vi "asap_spectrum.vi"() -> (6 "Raw signal":waveform(dbl)(graph))   [LabVIEW 2013]
uses:
  micron/labview/manipulator/squiggle/Host/i2c_interface.ctl
  micron/labview/manipulator/squiggle/Host/fpga_reference.ctl
  <vilib>/DAQmx/read.llb/DAQmx Read (Analog Wfm 1Chan NSamp).vi
  <vilib>/Analysis/2dsp.llb/Real FFT.vi
  <vilib>/Analysis/2dsp.llb/Inverse Real FFT.vi
  initialization/globals.vi
  <vilib>/DAQmx/miscellaneous.llb/DAQmx Fill In Error Info.vi
  <vilib>/Waveform/WDTOps.llb/WDT Get Waveform Subset DBL.vi
  <vilib>/Analysis/NI_AALPro.lvlib
panel:
  in  "Noise":bool
  out "Residue":waveform(dbl)(graph)
  out "Complex level":cdb=1.0+0.0i
  out "Nom phase":dbl format="%#_4p"
  out "0 dB level":dbl format="%#_4p"
  in  "Set level":bool
  out "Ref":cdb[][](array[numeric])
  in  "Min ampl":dbl=1e-05 format="%#_4p"
  in  "Hold":bool
  in  "Light":i32=-1
  in  "Normalize freq":bool=TRUE
  out "Output rate (s/s)":dbl
  out "Residue peaks":dbl[][](array[numeric]) format="%#_4p"
  in  "Set ref":bool
  out "Spectral peaks":dbl[][](array[numeric]) format="%#_4p"
  in  "Light enable":bool[](array[boolean])=[TRUE, TRUE, TRUE, TRUE, TRUE, TRUE]
  in  "Display blocks":i32=1
  in  "Skip":i32=1
  out "Acqusition rate (s/s)":dbl
  out "Raw Signal PSD":waveform(dbl)(graph) caption="FFT - (RMS)"
  in  "Updates/sec":sgl=5.0
  in  "stop":bool
  # "Ampl"
  # "phase"
  # "freq"
  # "f aliased"
  # "Ampl"
  # "phase"
  # "freq"
  # "f aliased"
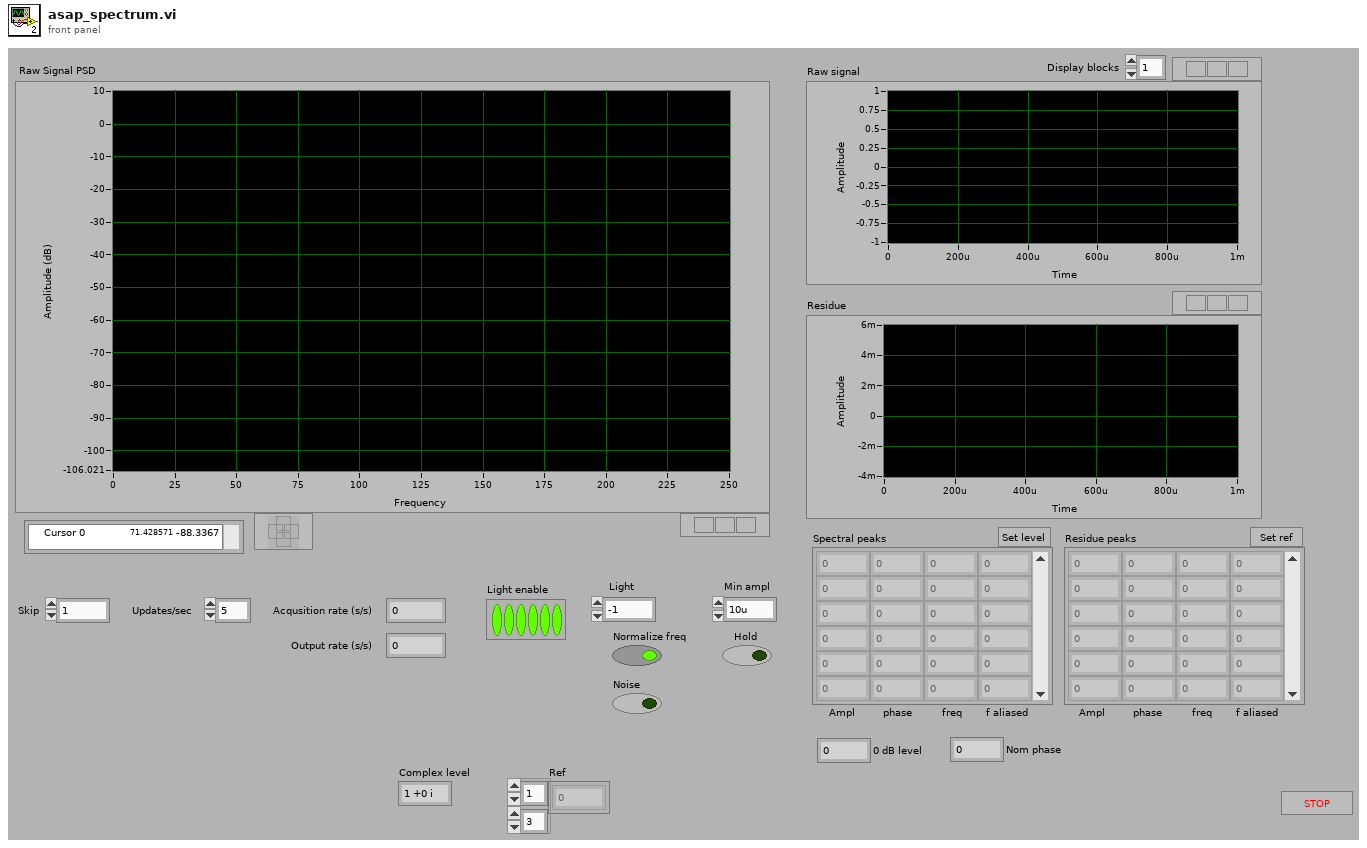
[diagram p1: front panel]
types:
  T1 = enum16{"ASAP/Trigger", "ASAP/Finder", "ASAP/Micron", "ASAP/Micron 2", "Micron 6DOF"}
  T2 = typedef "configuration.ctl" = cluster{"Calibration data":T3, "Block size":i32, "Tasks":cluster{"Analog Input":refnum<k21>, "Counters":refnum<k21>[], "Digital out":refnum<k21>}, "Light enables":bool[]}
  T3 = typedef "asap_calibration.ctl" = cluster{"T1":T4, "K1":T4, "T2":T4, "K2":T4, "Sensor LUT":sgl[][][][]}
  T4 = typedef "NI_Matrix.lvlib/RealMatrix.ctl" = dbl[][]
  T5 = cluster{"Analog Input":refnum<k21>, "Counters":refnum<k21>[], "Digital out":refnum<k21>}
  T6 = typedef "i2c_interface.ctl" = cluster{"FPGA VI Reference":T7}
  T7 = typedef "fpga_reference.ctl" = refnum<k20>
  T8 = cluster{"Fundamental":bool, "Harmonics":bool, "Noise":bool}
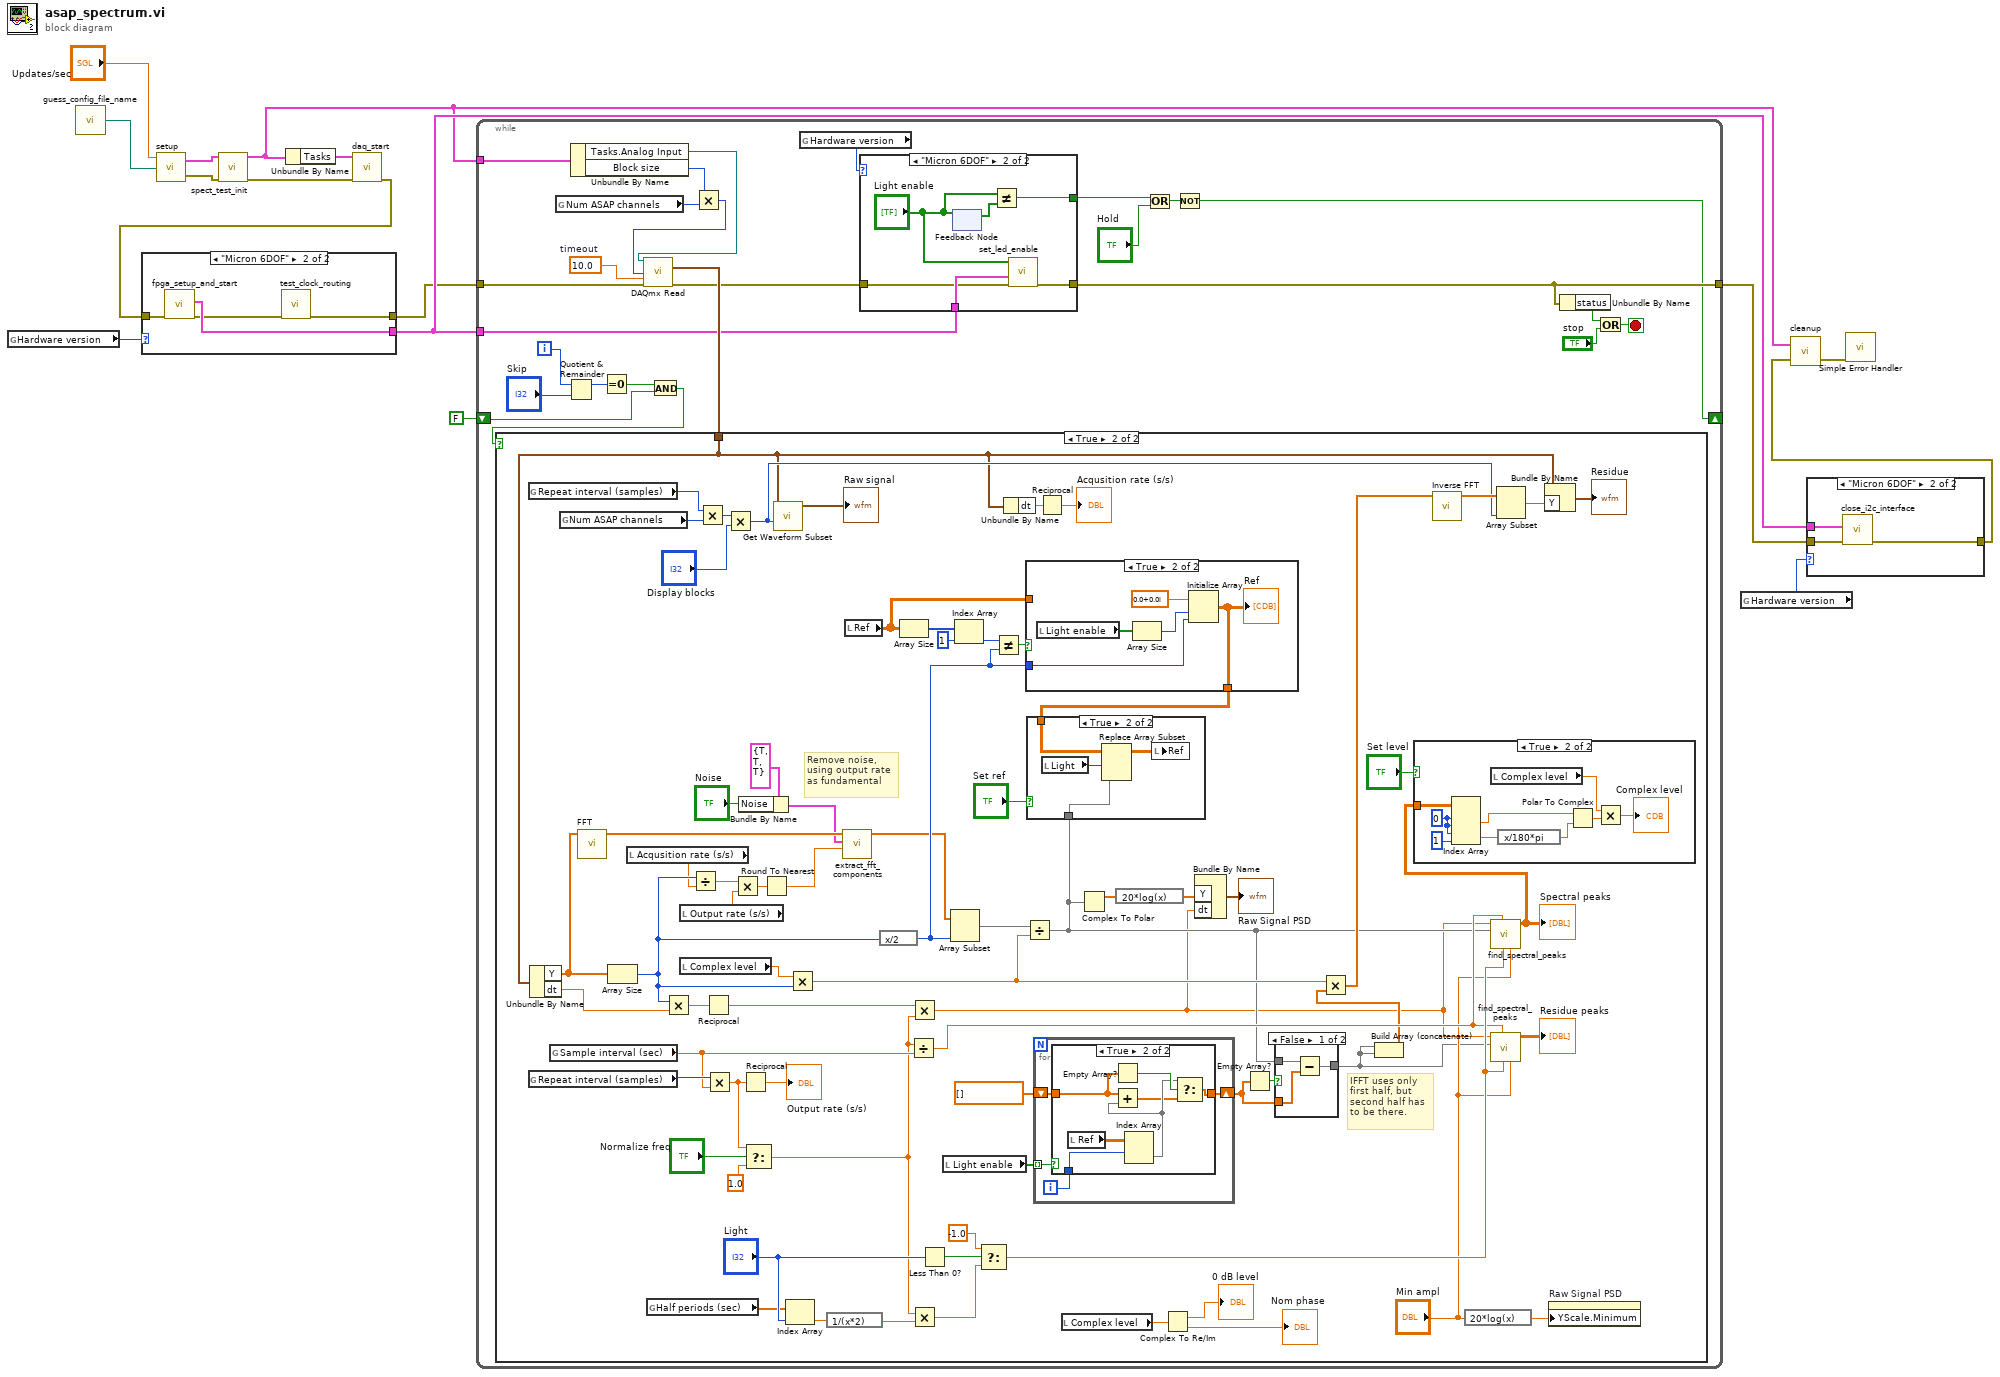
[diagram p0: block diagram]
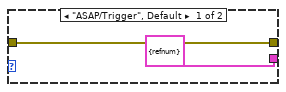
[diagram p3: hidden frame]
diagram:
  n1 = global read "globals.vi" "Hardware version"() -> (w10:T1)
  n2 = call "guess_config_file_name.vi"() -> ("config file path"=w16:path)
  n3 = call "setup.vi"("Calibration file name"=w16, "Updates/sec"="Updates/sec") -> ("error out"=w14:errorcluster, "Configuration"=w13:T2)  [unwired: 2 in]
  n4 = call "spect_test_init.vi"("error in"=w14, "Configuration in"=w13) -> ("error out"=w4:errorcluster, "Configuration out"=w5:T2)  [unwired: 8 in]
  n5 = Unbundle By Name(w5) -> ("Tasks"=w12:T5)
  n6 = call "daq_start.vi"("error in"=w4, "Tasks"=w12) -> ("error out"=w3:errorcluster)  [unwired: 9 out]
  n7 = case shown="\"Micron 6DOF\"" w10 {
    tunnel: w3 -> [w18 w22]
    tunnel: [w18 w19] -> w2
    tunnel: [T6 {"FPGA VI Reference"=refnum} ("I2C interface") w21] -> w6
    frame "ASAP/Trigger", Default {
    }
    frame "Micron 6DOF" {
      n8 = call "fpga_setup_and_start.vi"("error in"=w22) -> ("error out"=w20:errorcluster, "I2C interface"=w21:T6)  [unwired: 9 in]
      n9 = call "test_clock_routing.vi"("error in (no error)"=w20) -> ("error out"=w19:errorcluster)  [unwired: 10 in]
    }
  }
  n10 = while {
    tunnel: [w29] -> w8
    tunnel: w5 -> [w42]
    tunnel: w2 -> [w41]
    tunnel: w6 -> [w31]
    shift-right: [w23] -> _
    shift-left: FALSE ("x = 0?") -> [w27]
    i -> [w34]
    stop <- w43 stop-if-true
    w47 = 10.0  # timeout
    n11 = global read "globals.vi" "Num ASAP channels"() -> (w40:i32)
    n12 = Quotient & Remainder(x=w34, y="Skip") -> (x-y*floor(x/y)=w36:i32)  [unwired: 1 out]
    n13 = Unbundle By Name(w42) -> ("Tasks.Analog Input"=w46:refnum<k21>, "Block size"=w39:i32)
    n14 = Equal To 0?(x=w36) -> (x = 0?=w35:bool)
    n15 = Compound Arithmetic op=AND(w35, w27) -> (w33:bool)
    n16 = Multiply(x=w39, y=w40) -> (x*y=w38:i32)
    n17 = call-poly <vilib>:"DAQmx Read.vi"("task/channels in"=w46, "number of samples per channel"=w38, "timeout"=w47, "error in"=w41) -> ("data"=w37:waveform(dbl), "error out"=w30:errorcluster)  [unwired: 10 out]
    n18 = case shown="True" w33 {
      tunnel: w37 -> [_ w87]
      frame False {
      }
      frame True {
        # "Remove noise, using output rate as fundamental"
        # "IFFT uses only first half, but second half has to be there."
        n19 = global read "globals.vi" "Repeat interval (samples)"() -> (w124:i32)
        n20 = global read "globals.vi" "Repeat interval (samples)"() -> (w113:i32)
        n21 = Unbundle By Name(w87) -> ("Y"=w119:dbl[], "dt"=w118:dbl)
        n22 = global read "globals.vi" "Sample interval (sec)"() -> (w107:dbl)
        n23 = global read "globals.vi" "Num ASAP channels"() -> (w125:i32)
        n24 = call-poly <vilib>:"FFT.vi"("X"=w119) -> ("FFT {X}"=w66:cdb[])  [unwired: 9 in, 1 out]
        n25 = Array Size(array=w119) -> (size(s)=w64:i32)
        n26 = local read "Acqusition rate (s/s)"() -> (w63:dbl)
        n27 = global read "globals.vi" "Half periods (sec)"() -> (w103:dbl[])
        n28 = Multiply(x=w64, y=w118) -> (x*y=w117:dbl)
        n29 = local read "Output rate (s/s)"() -> (w56:dbl)
        n30 = local read "Complex level"() -> (w67:cdb)
        n31 = Divide(x=w64, y=w63) -> (x/y=w62:dbl)
        n32 = Multiply(x=w124, y=w125) -> (x*y=w123:i32)
        n33 = Reciprocal(x=w117) -> (1/x=w105:dbl)
        n34 = Multiply(x=w113, y=w107) -> (x*y=w109:dbl)
        n35 = Multiply(x=w123, y="Display blocks") -> (x*y=w89:i32)
        n36 = Multiply(x=w62, y=w56) -> (x*y=w58:dbl)
        n37 = Bundle By Name(cluster=T8 {"Fundamental"=TRUE, "Harmonics"=TRUE, "Noise"=TRUE} ("Components"), "Noise"="Noise") -> (w60:T8)
        n38 = Reciprocal(x=w109) -> (1/x=→"Output rate (s/s)":dbl)
        n39 = Select(t=w109, s="Normalize freq", f=1.0) -> (s? t:f=w99:dbl)
        n40 = Round To Nearest(number=w58) -> (nearest integer value=w57:dbl)
        n41 = call-poly <vilib>:"Get Waveform Subset.vi"("duration"=w89, "waveform in"=w87) -> ("waveform out"=→"Raw signal":waveform(dbl))  [unwired: 3 in, 4 out]
        n42 = Index Array(array=w103, index="Light") -> (element=w102:dbl)
        n43 = Multiply(x=w67, y=w64) -> (x*y=w82:cdb)
        n44 = expression code="1/(x*2)"(w102) -> (w101:dbl)
        n45 = call "extract_fft_components.vi"("Cycles in block"=w57, "Components"=w60, "FFT {X} in"=w66) -> ("FFT {X} out"=w65:cdb[])  [unwired: 8 in]
        n46 = local read "Ref"() -> (w77:cdb[][])
        n47 = expression code="x/2"(w64) -> (w69:i32)
        n48 = Array Size(array=w77) -> (size(s)=w80:i32[])
        n49 = Divide(x=w99, y=w107) -> (x/y=w106:dbl)
        n50 = Multiply(x=w105, y=w99) -> (x*y=w55:dbl)
        n51 = Multiply(x=w99, y=w101) -> (x*y=w100:dbl)
        n52 = Less Than 0?(x="Light") -> (x < 0?=w112:bool)
        n53 = local read "Light enable"() -> (w73:bool[])
        n54 = Array Subset(array=w65, length=w69) -> (w83:cdb[])  [unwired: 1 in]
        n55 = Index Array(array=w80, index=1) -> (element=w79:i32)
        n56 = Select(t=-1.0, s=w112, f=w100) -> (s? t:f=w111:dbl)
        n57 = Not Equal?(x=w79, y=w69) -> (x != y?=w78:bool)
        n58 = Unbundle By Name(w87) -> ("dt"=w128:dbl)
        n59 = case shown="True" w78 {
          tunnel: w69 -> [_ w151]
          tunnel: w77 -> [w149 _]
          tunnel: [w149 w150] -> w74
          frame False {
          }
          frame True {
            n60 = local read "Light enable"() -> (w153:bool[])
            n61 = Array Size(array=w153) -> (size(s)=w152:i32)
            n62 = Initialize Array(cdb 0.0+0.0i ("Complex level"), w152, w151) -> (w150:cdb[][])
            "Ref" <- w150
          }
        }
        n63 = Divide(x=w83, y=w82) -> (x/y=w75:cdb[])
        n64 = case shown="True" "Set ref" {
          tunnel: w75 -> [_ w146]
          tunnel: w74 -> [_ w148]
          frame False {
          }
          frame True {
            n65 = local read "Light"() -> (w147:i32)
            n66 = Replace Array Subset(array=w148, new element=w146, index (row)=w147) -> (w145:cdb[][])  [unwired: 1 in]
            n67 = local write "Ref"(w145) -> ()
          }
        }
        n68 = for {
          tunnel: w73 -> [w136] mode=indexing
          shift-right: [w133] -> w70
          shift-left: cdb[] [] ("x/y") -> [w134]
          i -> [w135]
          n69 = case shown="True" w136 {
            tunnel: w135 -> [_ w143]
            tunnel: w134 -> [w137 w141]
            tunnel: [w137 w138] -> w133
            frame False {
            }
            frame True {
              n70 = local read "Ref"() -> (w144:cdb[][])
              n71 = Empty Array?(array=w141) -> (empty?=w142:bool)
              n72 = Index Array(array=w144, index (row)=w143) -> (element=w140:cdb[])  [unwired: 1 in]
              n73 = Add(x=w141, y=w140) -> (x+y=w139:cdb[])
              n74 = Select(t=w140, s=w142, f=w139) -> (s? t:f=w138:cdb[])
            }
          }
        }
        n75 = Reciprocal(x=w128) -> (1/x=→"Acqusition rate (s/s)":dbl)
        n76 = local read "Complex level"() -> (w68:cdb)
        n77 = Complex To Polar(r * e^(i*theta)=w75) -> (r=w96:dbl[])  [unwired: 1 out]
        n78 = expression code="20*log(x)"(w96) -> (w120:dbl[])
        n79 = Complex To Re/Im(x + iy=w68) -> (x=→"0 dB level":dbl, y=→"Nom phase":dbl)
        n80 = Bundle By Name("Y"=w120, "dt"=w55) -> (→"Raw Signal PSD":waveform(dbl))  [unwired: 1 in]
        n81 = Empty Array?(array=w70) -> (empty?=w71:bool)
        n82 = case shown="False" w71 {
          tunnel: [w131 w132] -> w91
          tunnel: w75 -> [w130 w132]
          tunnel: w70 -> [w129 _]
          frame False {
            n83 = Subtract(x=w130, y=w129) -> (x-y=w131:cdb[])
          }
          frame True {
          }
        }
        n84 = Build Array (concatenate)(w91, w91) -> (w84:cdb[])
        n85 = Multiply(x=w82, y=w84) -> (x*y=w85:cdb[])
        n86 = call-poly <vilib>:"Inverse FFT.vi"("FFT {X}"=w85) -> ("X"=w90:dbl[])  [unwired: 9 in, 1 out]
        n87 = expression code="20*log(x)"("Min ampl") -> (w98:dbl)
        n88 = call "find_spectral_peaks.vi"("Min ampl"="Min ampl", "Freq filter"=w111, "Fs"=w106, "Complex Spectrum"=w75, "Freq res"=w55) -> ("Peaks"=w95:dbl[][])  [unwired: 6 in]
        "Spectral peaks" <- w95
        n89 = case shown="True" "Set level" {
          tunnel: w95 -> [_ w161]
          frame False {
          }
          frame True {
            w163 = 0 ("index (row)")
            n90 = Index Array(array=w161, index (row) #1=w163, index (col) #1=w163, index (row) #2=w163, index (col) #2=1 ("disabled index (col)")) -> (element #1=w159:dbl, element #2=w158:dbl)
            n91 = local read "Complex level"() -> (w155:cdb)
            n92 = expression code="x/180*pi"(w158) -> (w160:dbl)
            n93 = Polar To Complex(1:w160, 2:w159) -> (0:w157:cdb)
            n94 = Multiply(x=w155, y=w157) -> (x*y=→"Complex level":cdb)
          }
        }
        n95 = call "find_spectral_peaks.vi"("Min ampl"="Min ampl", "Freq filter"=w111, "Fs"=w106, "Complex Spectrum"=w91, "Freq res"=w55) -> ("Peaks"=→"Residue peaks":dbl[][])  [unwired: 6 in]
        n96 = Array Subset(array=w90, length=w89) -> (w88:dbl[])  [unwired: 1 in]
        n97 = Bundle By Name(cluster=w87, "Y"=w88) -> (→"Residue":waveform(dbl))
        n98 = property on="Raw Signal PSD" class="WFGraph (strict)"("YScale.Minimum"=w98) -> ()  [unwired: 2 in, 2 out]
      }
    }
    n99 = global read "globals.vi" "Hardware version"() -> (w32:T1)
    n100 = case shown="\"Micron 6DOF\"" w32 {
      tunnel: w31 -> [_ w54]
      tunnel: w30 -> [w48 w53]
      tunnel: [w48 w52] -> w29
      tunnel: [_ w49] -> w26
      frame "ASAP/Trigger", Default {
      }
      frame "Micron 6DOF" {
        n101 = feedback #1() -> (w51:bool[])  [unwired: 1 in]
        n102 = feedback-in #1("Light enable") -> ()
        n103 = Not Equal?(x="Light enable", y=w51) -> (x != y?=w49:bool)
        n104 = call "set_led_enable.vi"("error in"=w53, "I2C interface"=w54, "LED enables"="Light enable") -> ("error out"=w52:errorcluster)  [unwired: 8 in]
      }
    }
    n105 = Or(x=w26, y="Hold") -> (x .or. y?=w24:bool)
    n106 = Not(x=w24) -> (.not. x?=w23:bool)
    n107 = Unbundle By Name(w29) -> ("status"=w44:bool)
    n108 = Or(x=w44, y="stop") -> (x .or. y?=w43:bool)
  }
  n109 = global read "globals.vi" "Hardware version"() -> (w9:T1)
  n110 = case shown="\"Micron 6DOF\"" w9 {
    tunnel: [w164 w167] -> w7
    tunnel: w8 -> [w164 w166]
    tunnel: w6 -> [_ w165]
    frame "ASAP/Trigger", Default {
    }
    frame "Micron 6DOF" {
      n111 = call "close_i2c_interface.vi"("error in"=w166, "I2C interface"=w165) -> ("error out"=w167:errorcluster)  [unwired: 9 in]
    }
  }
  n112 = call "cleanup.vi"("error in"=w7, "Configuration"=w5) -> ("error out"=w15:errorcluster)  [unwired: 1 out]
  n113 = call <vilib>:"Simple Error Handler.vi"("error in (no error)"=w15) -> ()  [unwired: 1 in, 8 out]
